vi "BRig_RT_comm_tcp_write_RTwrite_adjustString.vi"(10 "input_packet":string) -> (2 "output_packet":string)   [LabVIEW 2014]
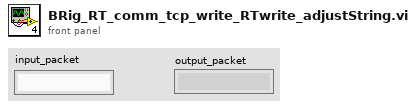
[diagram p1: front panel]
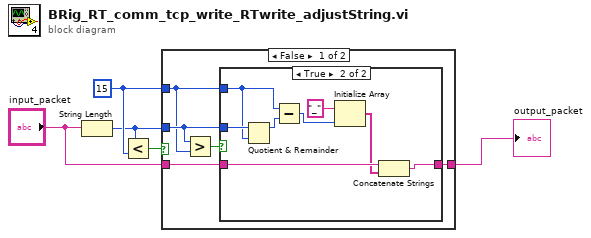
[diagram p0: block diagram]
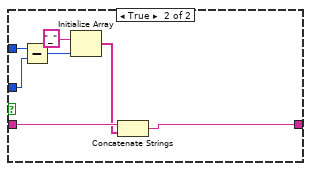
[diagram p3: hidden frame]
diagram:
  w5 = 15 ("y")
  n1 = String Length(string="input_packet") -> (length=w3:i32)
  n2 = Less?(x=w3, y=w5) -> (x < y?=w4:bool)
  n3 = case shown="False" w4 {
    tunnel: w5 -> [w7 w26]
    tunnel: w3 -> [w8 w25]
    tunnel: "input_packet" -> [w9 w21]
    tunnel: [w6 w22] -> w1
    frame False {
      n4 = Greater?(x=w8, y=w7) -> (0:w10:bool)
      n5 = case shown="True" w10 {
        tunnel: w9 -> [w11 w17]
        tunnel: w8 -> [_ w19]
        tunnel: w7 -> [_ w13]
        tunnel: [w11 w15] -> w6
        frame False {
        }
        frame True {
          n6 = Quotient & Remainder(x=w19, y=w13) -> (x-y*floor(x/y)=w14:i32)  [unwired: 1 out]
          n7 = Subtract(x=w13, y=w14) -> (x-y=w12:i32)
          n8 = Initialize Array("_", w12) -> (w16:string[])
          n9 = Concatenate Strings(w17, w16) -> (w15:string)
        }
      }
    }
    frame True {
      n10 = Subtract(x=w26, y=w25) -> (x-y=w24:i32)
      n11 = Initialize Array("_", w24) -> (w20:string[])
      n12 = Concatenate Strings(w21, w20) -> (w22:string)
    }
  }
  "output_packet" <- w1
